vi "Update Z Cursors.vi"(8 "error in":errorcluster, 11 "Analysis Graph in":refnum<class "Graph with Analysis Controls.lvclass">) -> (0 "error out":errorcluster)   [LabVIEW 2025, in "Graph with Analysis Controls.lvclass"]
uses:
  Graph with Analysis Controls.lvclass
  Series Graph/Graph with Series View.lvclass/Graph with Series View.ctl
  Graph with Analysis Controls.lvclass/Graph with Analysis Controls.ctl
  Base Graph/Base Graph.lvclass/Base Graph.ctl
  Base Graph/Get ROI Col-Row.vi
  Series Graph/Get Shots.vi
  Series Graph/Graph with Series View.lvclass
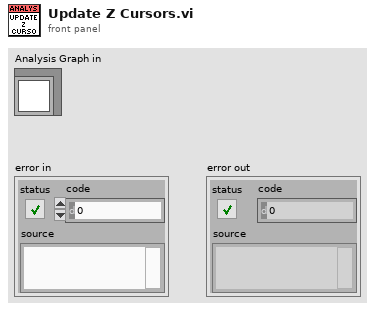
[diagram p1: front panel]
types:
  T1 = cluster{"ROI Col":cluster{"Index":u32, "Length":u32}, "ROI Row":cluster{"Index":u32, "Length":u32}, "ROI Z":cluster{"Index":u32, "Length":u32}}
  T2 = typedef "LVCursorListTypeDef.ctl" = cluster{"Name":string, "Color":u32, "Style":u8, "Point Style":u8, "Name Visible":bool, "Allow Drag":bool, "Cursor Mode":u32, "Plot":i32, "Index":i32, "Position":cluster{"X":dbl, "Y":dbl}, "X Scale":u32, "Y Scale":u32, "Watch Plots":i32[], "Watch All Plots":bool, "Plot Area":i32, "Label Offset":cluster{"X":dbl, "Y":dbl}}[]
  T3 = cluster{"Name":string, "Color":u32, "Style":u8, "Point Style":u8, "Name Visible":bool, "Allow Drag":bool, "Cursor Mode":u32, "Plot":i32, "Index":i32, "Position":cluster{"X":dbl, "Y":dbl}, "X Scale":u32, "Y Scale":u32, "Watch Plots":i32[], "Watch All Plots":bool, "Plot Area":i32, "Label Offset":cluster{"X":dbl, "Y":dbl}}
  T4 = cluster{"Name":string, "Color":u32, "Style":u8, "Point Style":u8, "Name Visible":bool, "Allow Drag":bool, "Cursor Mode":u32, "Plot":i32, "Index":i32, "Position":cluster{"X":dbl, "Y":dbl}, "X Scale":u32, "Y Scale":u32, "Watch Plots":i32[], "Watch All Plots":bool, "Plot Area":i32, "Label Offset":cluster{"X":dbl, "Y":dbl}}[]
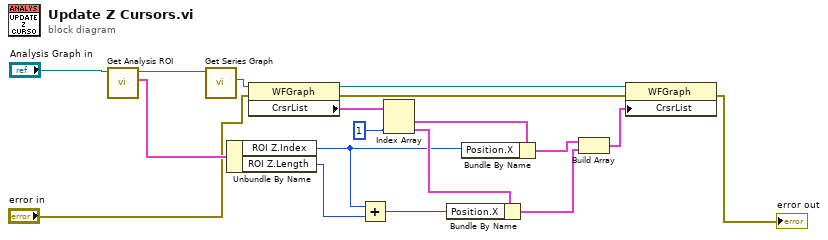
[diagram p0: block diagram]
diagram:
  n1 = call "Get Analysis ROI.vi"("Analysis Graph in"="Analysis Graph in") -> ("ROI Col Row Z"=w17:T1, "Analysis Graph out"=w3:refnum<class "Graph with Analysis Controls.lvclass">)  [unwired: 9 in]
  n2 = call "Get Series Graph.vi"("Series Graph in"=w3) -> ("Series Graph"=w16:refnum<vi>)  [unwired: 9 in, 1 out]
  n3 = Unbundle By Name(w17) -> ("ROI Z.Index"=w4:u32, "ROI Z.Length"=w11:u32)
  n4 = property class="WFGraph"(reference=w16, error in="error in") -> (reference out=w10:refnum<vi>, error out=w9:errorcluster, "CrsrList"=w15:T2)
  n5 = Add(x=w4, y=w11) -> (x+y=w5:u32)
  n6 = Index Array(array=w15, index #2=1 ("index")) -> (element #1=w13:T3, element #2=w12:T3)  [unwired: 1 in]
  n7 = Bundle By Name(cluster=w12, "Position.X"=w5) -> (w7:T3)
  n8 = Bundle By Name(cluster=w13, "Position.X"=w4) -> (w8:T3)
  n9 = Build Array(w8, w7) -> (w6:T4)
  n10 = property class="WFGraph"(reference=w10, error in=w9, "CrsrList"=w6) -> (error out=→"error out":errorcluster)  [unwired: 1 out]
